vi "annotate_segmentation.vi"() -> ()   [LabVIEW 2019]
uses:
  <vilib>/vision/NI_Vision_Development_Module.lvlib
panel:
  in  "images":string[](array[string])
  in  "class":T1(ring)
  out "error out":errorcluster
  in  "save label":bool
  in  "clear label":bool
  in  "segment":bool
  out "label":T2(plugin-control)
  in  "stop":bool
  out "original":T2(plugin-control)
  in  "error in (no error)":errorcluster
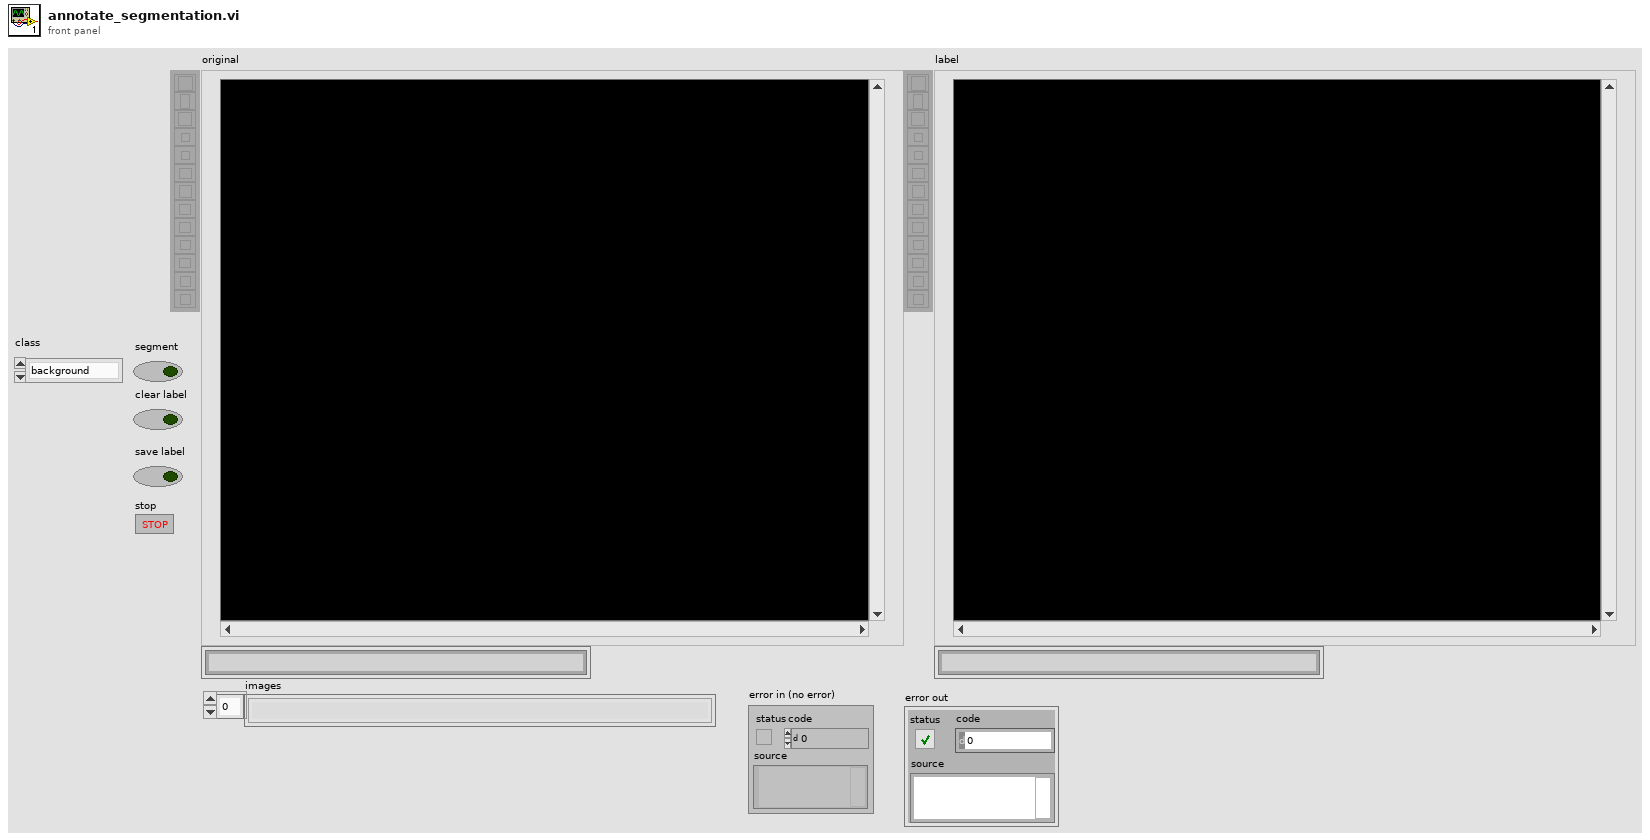
[diagram p1: front panel]
types:
  T1 = enum16{"background", "starling", "bluebird", "squirrel", "finch", "robin", "titmouse", "dove", "sparrow", "food"}
  T2 = typedef "IMAQ Image.ctl" = refnum<image>
  T3 = cluster{"Global Rectangle":i32[], "Contours":cluster{"Contour Type":u32, "ROI Type":u32, "Points":i32[]}[]}
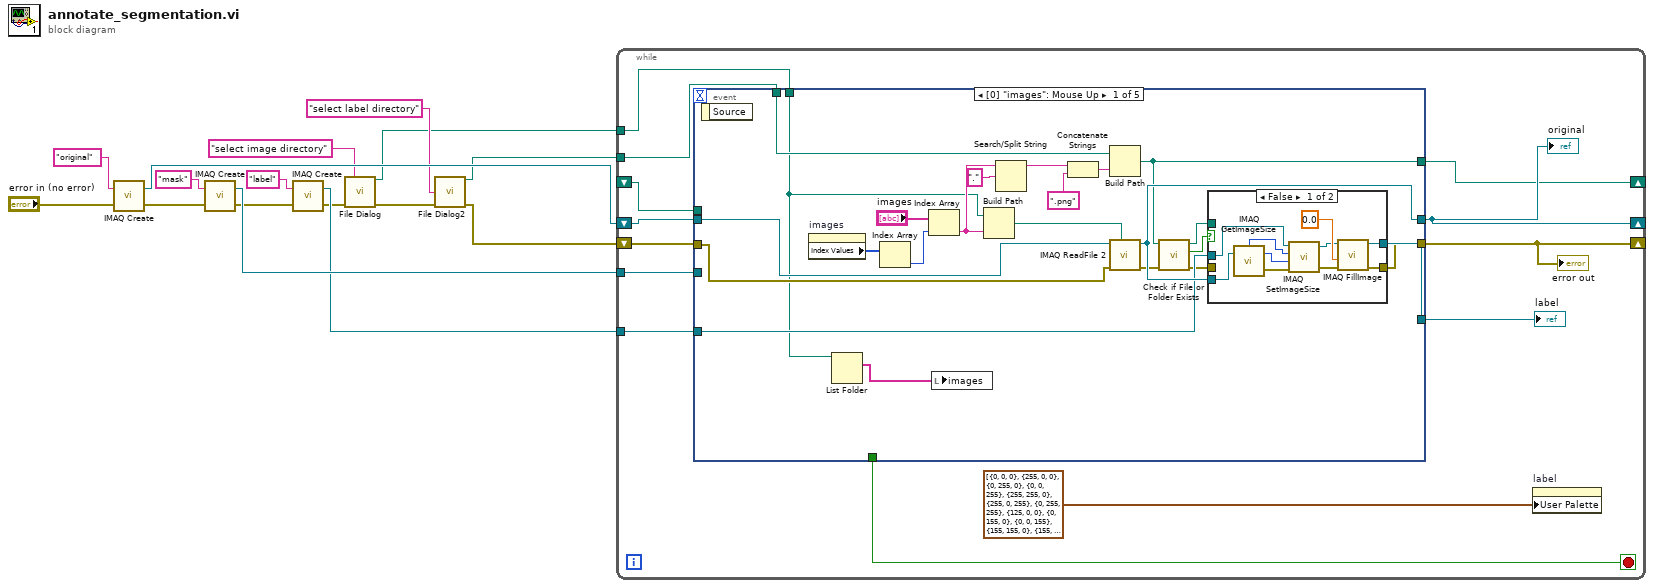
[diagram p0: block diagram]
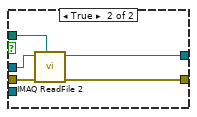
[diagram p2: hidden frame]
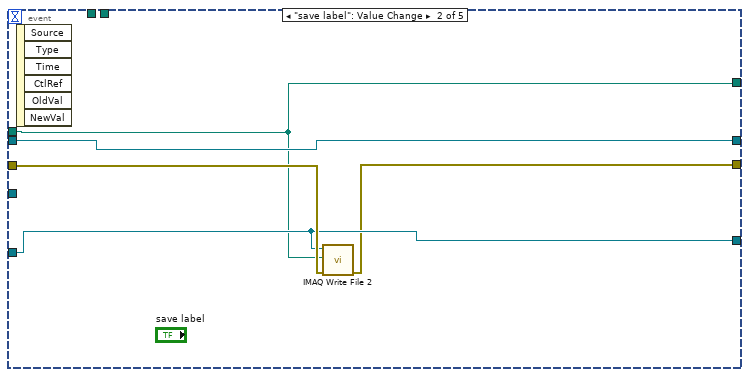
[diagram p3: hidden frame]
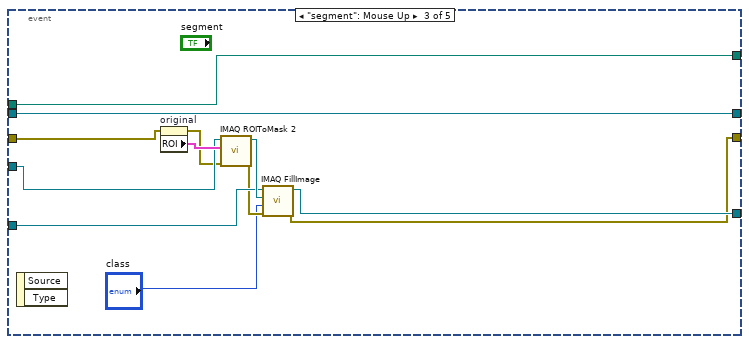
[diagram p4: hidden frame]
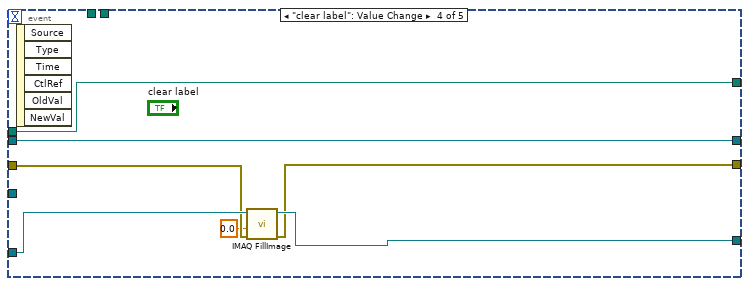
[diagram p5: hidden frame]
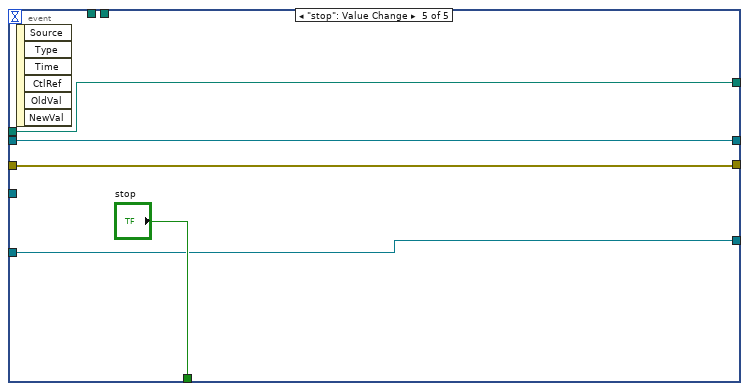
[diagram p6: hidden frame]
diagram:
  n1 = call "IMAQ Create"("Image Name"="original", "error in (no error)"="error in (no error)") -> ("New Image"=w15:T2, "error out"=w12:errorcluster)  [unwired: 3 in]
  n2 = call "IMAQ Create"("Image Name"="mask", "error in (no error)"=w12) -> ("New Image"=w11:T2, "error out"=w9:errorcluster)  [unwired: 3 in]
  n3 = call "IMAQ Create"("Image Name"="label", "error in (no error)"=w9) -> ("New Image"=w8:T2, "error out"=w7:errorcluster)  [unwired: 3 in]
  n4 = call "File Dialog"("prompt"="select image directory", "error in"=w7) -> ("selected path"=w2:path, "error out"=w5:errorcluster)  [unwired: 10 in, 2 out]
  n5 = call "File Dialog2"("default name"="select label directory" ("prompt"), "error in"=w5) -> ("selected path"=w1:path, "error out"=w4:errorcluster)  [unwired: 10 in, 2 out]
  n6 = while {
    shift-right: [w27] -> _
    shift-left: w4 -> [w29]
    shift-right: [w26] -> _
    shift-left: w15 -> [w28]
    tunnel: w11 -> [w24]
    tunnel: w8 -> [w23]
    tunnel: w2 -> [w20]
    tunnel: w1 -> [w18]
    shift-right: [w19] -> _
    shift-left: _ -> [w17]
    stop <- w25 stop-if-true
    n7 = event shown="[0] \"images\": Mouse Up" {
      selector: _ -> [_ _ _ _ _]
      dyn-events: _ -> [_ _ _ _ _]
      timeout: _ -> [_ _ _ _ _]
      tunnel: w29 -> [w52 w72 w78 w88 w94]
      tunnel: w28 -> [w51 w69 w84 w90 w93]
      tunnel: [w50 w69 w84 w90 w93] -> w26
      tunnel: [w42 w70 w75 w87 w94] -> w27
      tunnel: [_ _ _ _ "stop"] -> w25
      tunnel: w24 -> [_ _ w80 _ _]
      tunnel: w23 -> [w48 w71 w79 w89 w92]
      tunnel: [w49 w71 w81 w89 w92] -> w21
      tunnel: w20 -> [w31 _ _ _ _]
      tunnel: [w30 w68 w73 w85 w91] -> w19
      tunnel: w18 -> [w33 _ _ _ _]
      tunnel: w17 -> [_ w68 w73 w85 w91]
      event "images": Mouse Up {
        n8 = event-data() -> ()  [unwired: 1 in, 1 out]
        n9 = property on="images" class="Arr (strict)"() -> ("Index Values"=w38:u32[])  [unwired: 2 in, 2 out]
        n10 = List Folder(path=w31) -> (filenames=w32:string[])  [unwired: 3 in, 3 out]
        n11 = Index Array(array=w38) -> (element=w37:u32)  [unwired: 1 in]
        n12 = Index Array(array="images", index=w37) -> (element=w34:string)
        n13 = local write "images"(w32) -> ()
        n14 = Build Path(base path=w31, name or relative path=w34) -> (appended path=w35:path)
        n15 = Search/Split String(string=w34, search string/char (-)=".") -> (substring before match=w47:string)  [unwired: 1 in, 2 out]
        n16 = Concatenate Strings(w47, ".png" ("string")) -> (w46:string)
        n17 = Build Path(base path=w33, name or relative path=w46) -> (appended path=w30:path)
        n18 = call "IMAQ ReadFile 2"("File Path"=w35, "error in (no error)"=w52, "Image"=w51) -> ("error out"=w43:errorcluster, "Image Out"=w50:T2)  [unwired: 4 in, 3 out]
        n19 = call <vilib>:"Check if File or Folder Exists.vi"("error in (no error)"=w43, "path"=w30) -> ("error out"=w39:errorcluster, "file or folder exists?"=w41:bool, "dup path"=w40:path)  [unwired: 7 in]
        n20 = case shown="False" w41 {
          tunnel: w50 -> [w60 _]
          tunnel: [w53 w63] -> w49
          tunnel: w48 -> [w58 w67]
          tunnel: [w55 w64] -> w42
          tunnel: w40 -> [_ w66]
          tunnel: w39 -> [_ w65]
          frame False {
            n21 = call "IMAQ GetImageSize"("Image"=w60) -> ("Y Resolution"=w62:i32, "X Resolution"=w61:i32, "error out"=w59:errorcluster)  [unwired: 3 in]
            n22 = call "IMAQ SetImageSize"("error in (no error)"=w59, "Y Resolution"=w62, "X Resolution"=w61, "Image"=w58) -> ("error out"=w56:errorcluster, "Image Out"=w54:T2)  [unwired: 1 in]
            n23 = call "IMAQ FillImage"("error in (no error)"=w56, "Pixel Value (U8, U16, I16, Float)"=sgl 0.0, "Image"=w54) -> ("error out"=w55:errorcluster, "Image Out"=w53:T2)  [unwired: 7 in]
          }
          frame True {
            n24 = call "IMAQ ReadFile 2"("File Path"=w66, "error in (no error)"=w65, "Image"=w67) -> ("error out"=w64:errorcluster, "Image Out"=w63:T2)  [unwired: 4 in, 3 out]
          }
        }
      }
      event "save label": Value Change {
        n25 = event-data() -> ()  [unwired: 1 in, 6 out]
        n26 = call-poly "IMAQ Write File 2"("error in (no error)"=w72, "File Path"=w68, "Image"=w71) -> ("error out"=w70:errorcluster)  [unwired: 7 in, 1 out]
      }
      event "segment": Mouse Up {
        n27 = event-data() -> ()  [unwired: 1 in, 2 out]
        n28 = property on="original" class="ImageControl"(error in=w78) -> (error out=w77:errorcluster, "ROI"=w83:T3)  [unwired: 1 in, 1 out]
        n29 = call "IMAQ ROIToMask 2"("error in (no error)"=w77, "ROI Descriptor"=w83, "Image"=w80) -> ("error out"=w76:errorcluster, "Image Out"=w82:T2)  [unwired: 6 in, 1 out]
        n30 = call "IMAQ FillImage"("error in (no error)"=w76, "Pixel Value (U8, U16, I16, Float)"="class", "Image Mask"=w82, "Image"=w79) -> ("error out"=w75:errorcluster, "Image Out"=w81:T2)  [unwired: 6 in]
      }
      event "clear label": Value Change {
        n31 = event-data() -> ()  [unwired: 1 in, 6 out]
        n32 = call "IMAQ FillImage"("error in (no error)"=w88, "Pixel Value (U8, U16, I16, Float)"=sgl 0.0, "Image"=w89) -> ("error out"=w87:errorcluster)  [unwired: 7 in, 1 out]
      }
      event "stop": Value Change {
        n33 = event-data() -> ()  [unwired: 1 in, 6 out]
      }
    }
    "original" <- w26
    "label" <- w21
    "error out" <- w27
    n34 = property on="label" class="ImageControl"("User Palette"=cluster{"Red":u8, "Green":u8, "Blue":u8}[] [{"Red"=0, "Green"=0, "Blue"=0}, {"Red"=255, "Green"=0, "Blue"=0}, {"Red"=0, "Green"=255, "Blue"=0}, {"Red"=0, "Green"=0, "Blue"=255}, {"Red"=255, "Green"=255, "Blue"=0}, {"Red"=255, "Green"=0, "Blue"=255}, {"Red"=0, "Green"=255, "Blue"=255}, {"Red"=125, "Green"=0, "Blue"=0}, {"Red"=0, "Green"=155, "Blue"=0}, {"Red"=0, "Green"=0, "Blue"=155}, {"Red"=155, "Green"=155, "Blue"=0}, {"Red"=155, "Green"=0, "Blue"=155}, {"Red"=0, "Green"=155, "Blue"=155}, {"Red"=255, "Green"=255, "Blue"=255}, {"Red"=155, "Green"=155, "Blue"=155}] ("Palette:User Palette")) -> ()  [unwired: 2 in, 2 out]
  }
